vi "Gravação_de_Arquivo.vi"() -> ()   [LabVIEW 2012]
panel:
  in  "file path (use dialog)":path
  in  "text":string
  in  "OK Button":bool
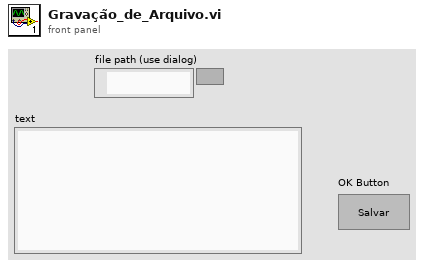
[diagram p1: front panel]
types:
  T1 = enum16{"open", "replace", "create", "open or create", "replace or create", "replace or create with confirmation"}
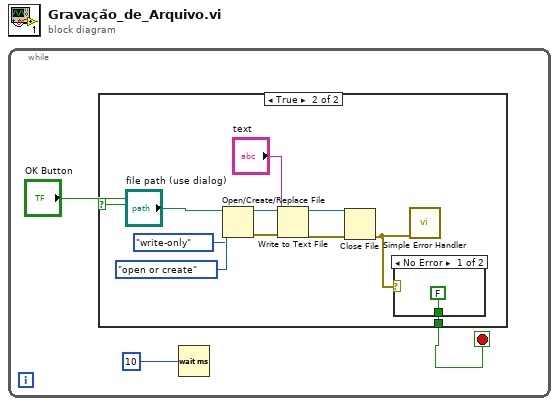
[diagram p0: block diagram]
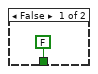
[diagram p2: hidden frame]
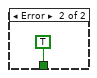
[diagram p3: hidden frame]
diagram:
  n1 = while {
    stop <- w1 stop-if-true
    n2 = case shown="True" "OK Button" {
      tunnel: [FALSE w6] -> w1
      frame False {
      }
      frame True {
        n3 = Open/Create/Replace File(file path (use dialog)="file path (use dialog)", operation (0:open)=T1."open or create", access (0:read/write)=enum16{"read/write", "read-only", "write-only"}."write-only") -> (refnum out=w11:refnum<file>, error out=w14:errorcluster)  [unwired: 3 in, 1 out]
        n4 = Write to Text File(file (use dialog)=w11, text="text", error in=w14) -> (refnum out=w12:refnum<file>, error out=w13:errorcluster)  [unwired: 1 in, 1 out]
        n5 = Close File(refnum=w12, error in=w13) -> (error out=w10:errorcluster)  [unwired: 1 out]
        n6 = case shown="No Error" w10 {
          tunnel: [FALSE TRUE] -> w6
          frame No Error {
          }
          frame Error {
          }
        }
        n7 = call <vilib>:"Simple Error Handler.vi"("error in (no error)"=w10) -> ()  [unwired: 4 in, 5 out]
      }
    }
    n8 = Wait (ms)(milliseconds to wait=10) -> ()  [unwired: 1 out]
  }
